vi "Parse Response JSON.vi"(8 "error in (no error)":errorcluster, 10 "Response JSON":string, 11 "RGetSourceScreenshot in":refnum<class "RGetSourceScreenshot.lvclass">) -> (0 "error out":errorcluster, 3 "RGetSourceScreenshot out":refnum<class "RGetSourceScreenshot.lvclass">)   [LabVIEW 2020, in "obs-websocket.lvlib" / "RGetSourceScreenshot.lvclass"]
uses:
  RGetSourceScreenshot.lvclass
  RGetSourceScreenshot.lvclass/RGetSourceScreenshot.ctl
  lv-web-crypto/lv-base64/Base64.lvlib
  <vilib>/wsapi/NI_WebServices.lvlib
  adbed530-4c55-4512-aa71-fae98708a437.vi
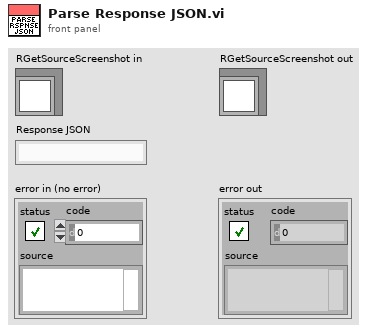
[diagram p1: front panel]
types:
  T1 = typedef "imagedata.ctl" = cluster{"image type":i32, "image depth":i32, "image":u8[], "mask":u8[], "colors":u32[], "Rectangle":cluster{"left":i16, "top":i16, "right":i16, "bottom":i16}}
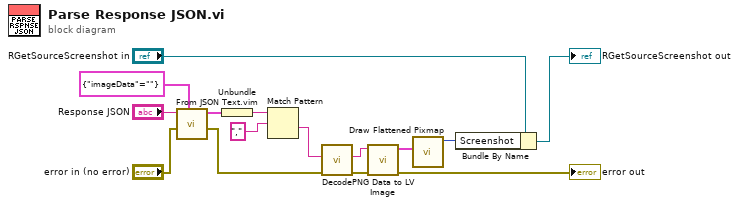
[diagram p0: block diagram]
diagram:
  n1 = call "From JSON Text.vim"("Data Type and Default Value"=cluster{"imageData":string} {"imageData"=""}, "error in (no error)"="error in (no error)", "JSON"="Response JSON") -> ("error out"=w15:errorcluster, "Data out"=w3:cluster{"imageData":string})  [unwired: 7 in]
  n2 = Unbundle(w3) -> ("imageData"=w2:string)
  n3 = Match Pattern(string=w2, regular expression=",") -> (after substring=w6:string)  [unwired: 1 in, 3 out]
  n4 = call "Decode.vi"("error in (no error)"=w15, "string in (base64-encoded)"=w6) -> ("error out"=w8:errorcluster, "string out (decoded)"=w12:string)  [unwired: 8 in]
  n5 = call <vilib>:"PNG Data to LV Image.vi"("error in (no error)"=w8, "png data"=w12) -> ("error out"=→"error out":errorcluster, "image data"=w11:T1)  [unwired: 8 in]
  n6 = call <vilib>:"Draw Flattened Pixmap.vi"("image data"=w11) -> ("new picture"=w9:picture)  [unwired: 8 in]
  n7 = Bundle By Name(cluster="RGetSourceScreenshot in", "Screenshot"=w9) -> (→"RGetSourceScreenshot out":refnum<class "RGetSourceScreenshot.lvclass">)
